vi "publish stucture.vi"(8 "Error In":errorcluster, 10 "OPC UA server refnum in":refnum<k21>, 11 "DOM document in":refnum<k20>) -> (0 "Error Out":errorcluster, 2 "OPC UA server refnum out":refnum<k21>, 3 "DOM document out":refnum<k20>)   [LabVIEW 2013, in "CreateOPCUAServerAuto.lvlib"]
uses:
  CreateOPCUAServerAuto.lvlib
  <vilib>/xml/Close Reference(Node).vi
  <resource>/objmgr/DOMUserDefRef.rc
  <vilib>/xml/NI_XML.lvlib
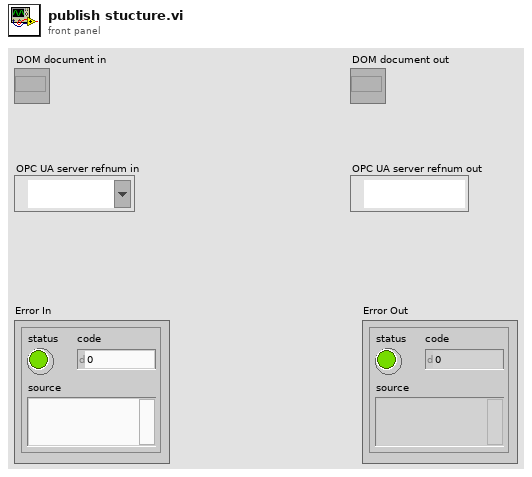
[diagram p1: front panel]
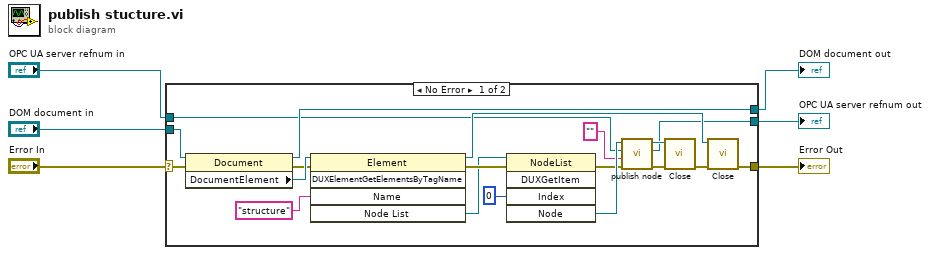
[diagram p0: block diagram]
diagram:
  n1 = case shown="No Error" "Error In" {
    selector: "Error In" -> [w25 w28]
    tunnel: [w20 w28] -> w6
    tunnel: "DOM document in" -> [w24 w27]
    tunnel: [w23 w27] -> w3
    tunnel: "OPC UA server refnum in" -> [w8 w26]
    tunnel: [w7 w26] -> w1
    frame No Error {
      n2 = property class="Document"(reference=w24, error in=w25) -> (reference out=w23:refnum<k20>, error out=w21:errorcluster, "DocumentElement"=w22:refnum<k20>)
      n3 = invoke class="Element" method="DUXElementGetElementsByTagName"(reference=w22, error in=w21, "Name"="structure") -> (reference out=w16:refnum<k20>, error out=w18:errorcluster, "Node List"=w15:refnum<k20>)  [unwired: 2 in, 2 out]
      n4 = invoke class="NodeList" method="DUXGetItem"(reference=w15, error in=w18, "Index"=0) -> (error out=w13:errorcluster, "Node"=w14:refnum<k20>)  [unwired: 2 in, 3 out]
      n5 = call "publish node.vi"("Error In"=w13, "parent opcua path"="", "OPC UA server refnum in"=w8, "DOM node"=w14) -> ("Error Out"=w10:errorcluster, "OPC UA server refnum out"=w7:refnum<k21>, "DOM node (dup)"=w11:refnum<k20>)  [unwired: 5 in]
      n6 = call-poly <vilib>:"Close.vi"("error in (no error)"=w10, "node"=w11) -> ("error out"=w9:errorcluster)  [unwired: 7 out]
      n7 = call-poly <vilib>:"Close.vi"("error in (no error)"=w9, "node"=w16) -> ("error out"=w20:errorcluster)  [unwired: 7 out]
    }
    frame Error {
    }
  }
  "Error Out" <- w6
  "DOM document out" <- w3
  "OPC UA server refnum out" <- w1
